vi "createEvents.vi"(8 "error in (no error)":errorcluster, 11 "PubSubDataEvent in":refnum<class "PubSubDataEvent.lvclass">) -> (0 "error out":errorcluster, 3 "PubSubDataEvent out":refnum<class "PubSubDataEvent.lvclass">)   [LabVIEW 2015, in "PubSubDataEvent.lvclass"]
uses:
  PubSubDataEvent.lvclass
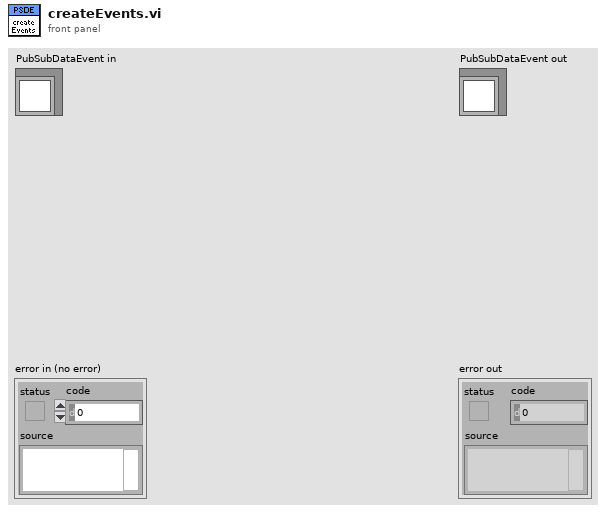
[diagram p1: front panel]
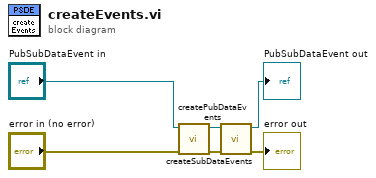
[diagram p0: block diagram]
diagram:
  n1 = call "createPubDataEvents.vi"("error in (no error)"="error in (no error)", "PubSubDataEvent in"="PubSubDataEvent in") -> ("error out"=w4:errorcluster, "PubSubDataEvent out"=w6:refnum<class "PubSubDataEvent.lvclass">)  [unwired: 8 in]
  n2 = call "createSubDataEvents.vi"("error in (no error)"=w4, "PubSubDataEvent in"=w6) -> ("error out"=→"error out":errorcluster, "PubSubDataEvent out"=→"PubSubDataEvent out":refnum<class "PubSubDataEvent.lvclass">)  [unwired: 8 in]
